vi "Begin.vi"(8 "error in (no error)":errorcluster, 10 "Settings":variant, 11 "Drive in":refnum<class "Drive.lvclass">) -> (0 "error out":errorcluster, 3 "Drive out":refnum<class "Drive.lvclass">)   [LabVIEW 2019, in "DriveOld.lvlib" / "Drive.lvclass"]
doc: "This VI holds the begin code"
uses:
  Drive.lvclass
  Drive.lvclass/Drive.ctl
  Write Drive Velocity Low Gear.vi
  Write Drive Velocity High Gear.vi
  Write Drive Motion Magic Primary Low Gear.vi
  Write Drive Motion Magic Primary High Gear.vi
  Write Drive Motion Magic Secondary High Gear.vi
  Write Drive Motion Magic Secondary Low Gear.vi
  Write Motion Magic Constants.vi
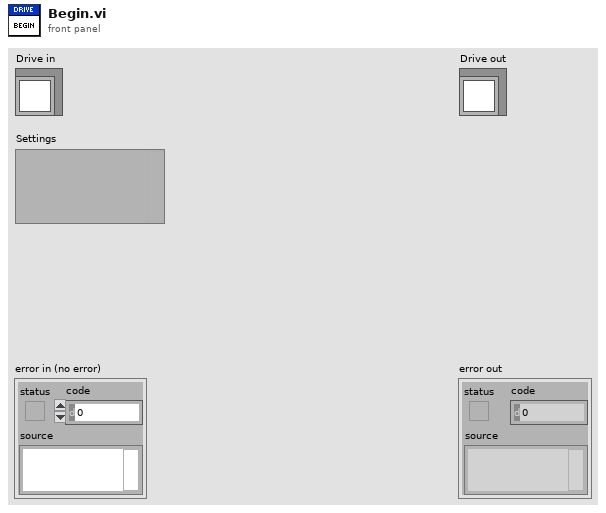
[diagram p1: front panel]
types:
  T1 = typedef "CTRE_Phoenix_MotorControl_SlotStructure.ctl" = cluster{"P":dbl, "I":dbl, "D":dbl, "F":dbl, "integralZone":dbl, "allowableClosedLoopError":i32, "maxIntegralAccumulator":dbl, "closedLoopPeakOutput":dbl, "closedLoopPeriod":i32}
  T2 = typedef "DriveOld.lvlib/Drive.lvclass/Drive Sensor Data.ctl" = cluster{"Drive Right Invert":bool, "Drive Right Sensor Phase":bool, "Drive Left Invert":bool, "Drive Left Sensor Phase":bool}
  T3 = typedef "DriveOld.lvlib/Drive.lvclass/Motion Magic Constants.ctl" = cluster{"Low Gear Max Velocity":u32, "High Gear Max Velocity":u32, "Motion Magic Low Gear Max Velocity":u32, "Motion Magic Low Gear Max Acceleration":u32, "Motion Magic High Gear Max Velocity":u32, "Motion Magic High Gear Max Acceleration":u32}
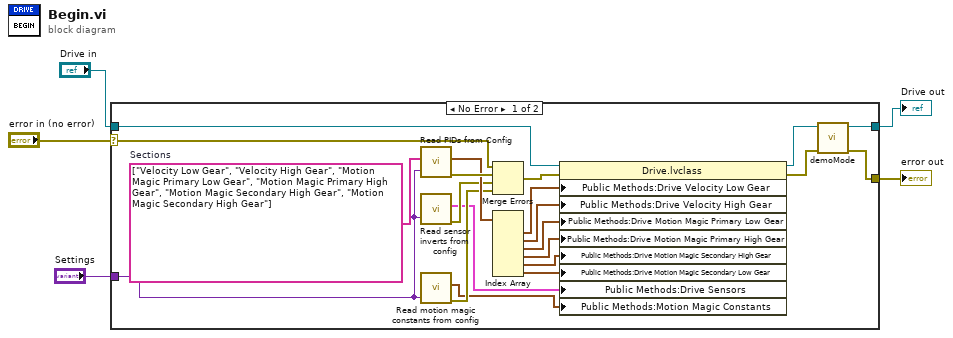
[diagram p0: block diagram]
diagram:
  n1 = case shown="No Error" "error in (no error)" {
    selector: "error in (no error)" -> [w24 w28]
    tunnel: [w8 w28] -> w4
    tunnel: [w9 w27] -> w2
    tunnel: "Drive in" -> [w26 w27]
    tunnel: "Settings" -> [w6 _]
    frame No Error {
      w22 = string[] ["Velocity Low Gear", "Velocity High Gear", "Motion Magic Primary Low Gear", "Motion Magic Primary High Gear", "Motion Magic Secondary High Gear", "Motion Magic Secondary High Gear"]  # Sections
      n2 = call "Read PIDs from Config.vi"("keys"=w22, "Settings"=w6) -> ("error out"=w23:errorcluster, "Array"=w21:T1[])  [unwired: 7 in, 1 out]
      n3 = call "Read sensor inverts from config.vi"("Settings"=w6) -> ("error out"=w13:errorcluster, "Drive Sensors"=w12:T2)  [unwired: 8 in, 1 out]
      n4 = call "Read motion magic constants from config.vi"("Settings"=w6) -> ("error out"=w14:errorcluster, "Motion Magic Constants"=w11:T3)  [unwired: 8 in, 1 out]
      n5 = Merge Errors(w24, w23, w13, w14) -> (w25:errorcluster)
      n6 = Index Array(array=w21) -> (element #1=w20:T1, element #2=w19:T1, element #3=w18:T1, element #4=w17:T1, element #5=w16:T1, element #6=w15:T1)  [unwired: 6 in]
      n7 = property class="Drive.lvclass"(reference=w26, error in=w25, "Public Methods:Drive Velocity Low Gear"=w20, "Public Methods:Drive Velocity High Gear"=w19, "Public Methods:Drive Motion Magic Primary Low Gear"=w18, "Public Methods:Drive Motion Magic Primary High Gear"=w17, "Public Methods:Drive Motion Magic Secondary High Gear"=w16, "Public Methods:Drive Motion Magic Secondary Low Gear"=w15, "Public Methods:Drive Sensors"=w12, "Public Methods:Motion Magic Constants"=w11) -> (reference out=w10:refnum<class "Drive.lvclass">, error out=w7:errorcluster)
      n8 = call "demoMode.vi"("error in (no error)"=w7, "Pod Drive in"=w10) -> ("error out"=w8:errorcluster, "Pod Drive out"=w9:refnum<class "Drive.lvclass">)  [unwired: 8 in]
    }
    frame Error {
    }
  }
  "error out" <- w4
  "Drive out" <- w2
